vi "GOMDBTS2048 spectral Get Integration Time Range Inus.vi"(8 "error in (no error)":errorcluster, 11 "handle":i32) -> (0 "error out":errorcluster, 1 "function return":i32, 2 "max":i32, 3 "min":i32)   [LabVIEW 2015, in "GOMDBTS2048.lvlib"]
doc: "GOBTS2048DLL int __stdcall GOMDBTS2048_spectralGetIntegrationTimeRangeInus(int handle, int* min, int* max);"
uses:
  GOMDBTS2048.lvlib
  runtime/GOMDBTS2048.dll
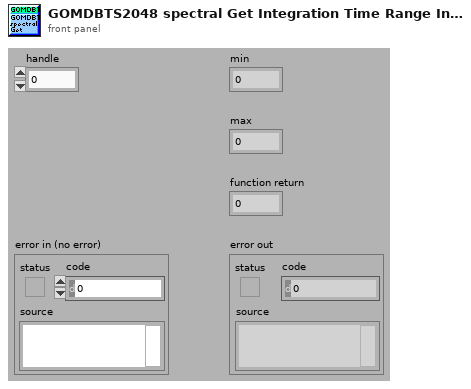
[diagram p1: front panel]
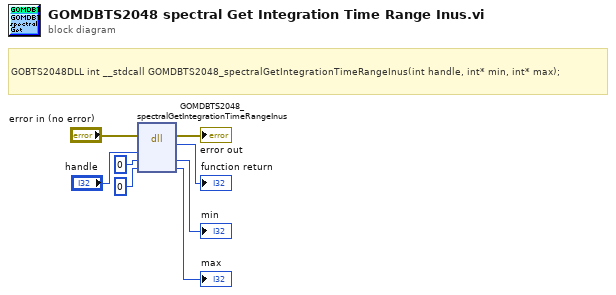
[diagram p0: block diagram]
diagram:
  # "GOBTS2048DLL int __stdcall GOMDBTS2048_spectralGetIntegrationTimeRangeInus(int handle, int* min, int* max);"
  n1 = dll-call lib="C:/Users/rkoch/Documents/GO_Library/runtime/GOMDBTS2048.*" fn="GOMDBTS2048_spectralGetIntegrationTimeRangeInus"(error in="error in (no error)", "handle"="handle", "min"=0, "max"=0) -> (error out=→"error out":errorcluster, →"function return":i32, "min"=→"min":i32, "max"=→"max":i32)  [unwired: 3 in, 1 out]
